vi "direct_ads_vol_A_WRho.vi"(8 "Error (Input)":errorcluster, 9 "Saturated liquid density of adsorpt rho_l in kg/m3 (Input)":dbl, 10 "Volumetric loading W in m3/kg (Input)":dbl, 11 "WorkingPair (Input)":T1={"no_iso"=1, "no_p_sat"=1, "path_db"="D:\\Driesel\\SorpLibLocal\\LabVIEW_wrapper\\data\\json\\sorpproplib_minimalExample.json", "wp_as"="silicagel", "wp_st"="123", "wp_iso"="DubininArctan1", "wp_rf"="water", "rf_rhol"="SaturatedLiquidDensity_EoS1", "no_rhol"=1, "rf_psat"="VaporPressure_EoS1"}) -> (0 "Error (Output)":errorcluster caption="Error(Output)", 3 "Equilibrium adsorption potential A in J/mol (Output)":dbl)   [LabVIEW 2017]
doc: "direct_ads_vol_A_WRho:\n * ----------------------\n *\n * Calculates equilibrium adsorption potential A in J/mol depending on\n * equilibrium volumetric loading W in m³/kg and saturated liquid density of\n * adsorpt rho_l in kg/m3.\n *\n * Parameters:\n * -----------\n * double W_m3kg:\n * Equilibrium volumetric loading W in m³/kg.\n * double rho_l_kgm3:\n * Saturated liquid density of adsorpt rho_l in kg/m3.\n *\n * const char *path_db:\n * Path to database.\n * const char *wp_as:\n * Name of sorbent.\n * const char *wp_st:\n * Name of sub-type of sorbent.\n * const char *wp_rf:\n * Name of refrigerant.\n * const char *wp_iso:\n * Name of isotherm.\n * int no_iso:\n * ID of isotherm (i.e. when more than one isotherm is available)\n * const char *rf_psat:\n * Name of calculation approach for vapor pressure.\n * int no_p_sat:\n * ID of vapor pressure equation (i.e. when more than one equation is\n * available)\n * const char *rf_rhol:\n * Name of calculation approach for liquid density.\n * int no_rhol:\n * ID of liquid density equation (i.e. when more than one equation is\n * available)\n *\n * Returns:\n * --------\n * double:\n * Equilibrium adsorption potential A in J/mol.\n *\n * Remarks:\n * --------\n * This function is only valid for isotherm models based on the volumetric\n * approach.\n * Saturated liquid density of adsorpt is required to calculate volumetric\n * loading from characteristic curve in m3/kg when coefficients would directly\n * return loading w in kg/kg.\n *\n * History:\n * --------\n * 07/07/2021, by Jannik Driesel (supervised by Mirko Engelpracht):\n * First implementation."
uses:
  data/win32bit/libsorpPropLib.dll
panel:
  # "Path to database"
  # "Name of sorbent"
  # "Name of sub-type of sorbent"
  # "Name of refrigerant"
  # "Name of isotherm"
  # "ID of isotherm"
  # "Name of calculation approach for vapor pressure"
  # "ID of vapor pressure equation"
  # "Name of calculation approach for liquid density"
  # "ID of liquid density equation"
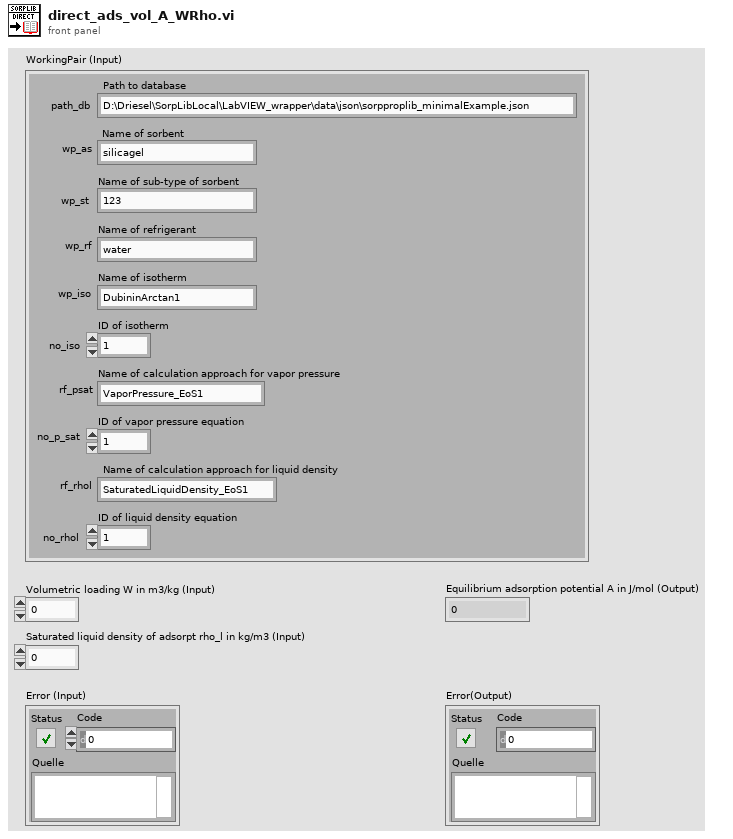
[diagram p1: front panel]
types:
  T1 = cluster{"no_iso":i32, "no_p_sat":i32, "path_db":string, "wp_as":string, "wp_st":string, "wp_iso":string, "wp_rf":string, "rf_rhol":string, "no_rhol":i32, "rf_psat":string}
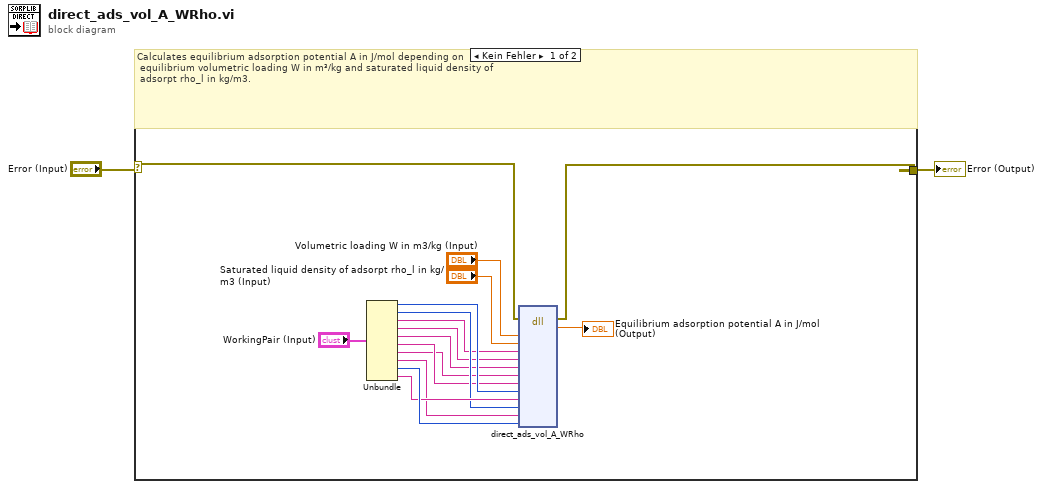
[diagram p0: block diagram]
diagram:
  n1 = case shown="Kein Fehler" "Error (Input)" {
    selector: "Error (Input)" -> [w6 w19]
    tunnel: [w5 w19] -> w1
    frame No Error {
      # "Calculates equilibrium adsorption potential A in J/mol depending on\n equilibrium volumetric loading W in m³/kg and saturated liquid density of\n adsorpt rho_l in kg/m3."
      n2 = Unbundle("WorkingPair (Input)") -> ("no_iso"=w14:i32, "no_p_sat"=w15:i32, "path_db"=w8:string, "wp_as"=w9:string, "wp_st"=w10:string, "wp_iso"=w12:string, "wp_rf"=w11:string, "rf_rhol"=w13:string, "no_rhol"=w17:i32, "rf_psat"=w16:string)
      n3 = dll-call lib="D:/Driesel/SorpLibLocal/LabVIEW_wrapper/data/win32bit/libsorpPropLib.dll" fn="direct_ads_vol_A_WRho"(error in=w6, "W_m3kg"="Volumetric loading W in m3/kg (Input)", "rho_1_kgm3"="Saturated liquid density of adsorpt rho_l in kg/m3 (Input)", "path_db"=w8, "wp_as"=w9, "wp_st"=w10, "wp_rf"=w11, "wp_iso"=w12, "no_iso"=w14, "rf_psat"=w16, "no_p_sat"=w15, "rf_rhol"=w13, "no_rhol"=w17) -> (error out=w5:errorcluster, "A_Jmol"=→"Equilibrium adsorption potential A in J/mol (Output)":dbl)  [unwired: 14 in, 1 out]
    }
    frame Error {
      # "Error - No calculations"
    }
  }
  "Error (Output)" <- w1
